vi "demo.vi"() -> ()   [LabVIEW 2016]
uses:
  test/apis/Stimulus/Helper/Helper-SubPanel/Helper-SubPanel.vi
  main/apis/Stimulus/ValueSignalByPathString.vi
  <vilib>/addons/_JKI Toolkits/Caraya/classes/Test/Test.lvclass
  test/apis/Stimulus/test_ValueSignal.lvlib
panel:
  out "error out":errorcluster
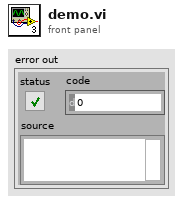
[diagram p1: front panel]
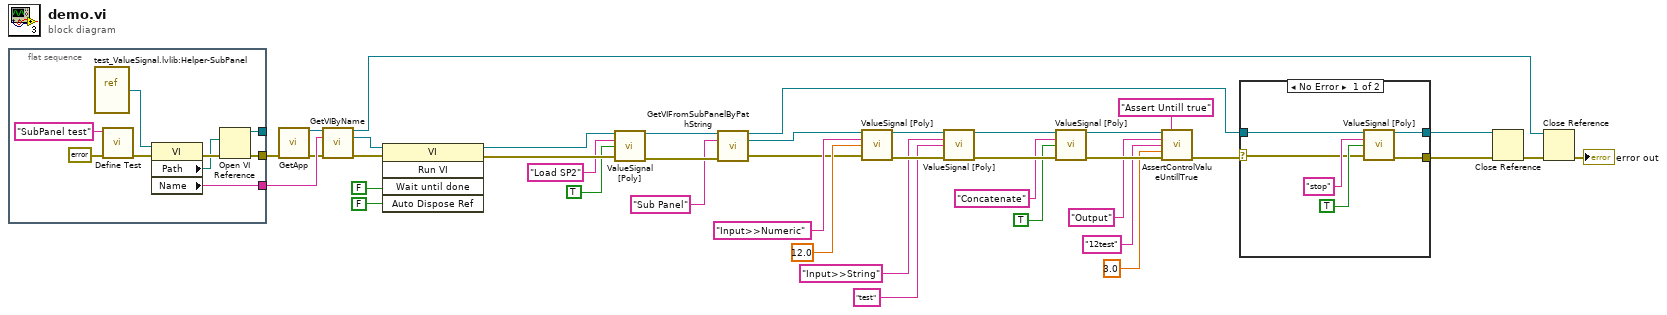
[diagram p0: block diagram]
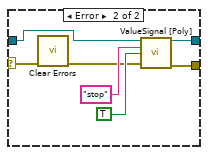
[diagram p2: hidden frame]
diagram:
  n1 = flat-sequence {
    tunnel: [w45] -> w39
    tunnel: [w44] -> _
    tunnel: [w42] -> w38
    frame #0 {
      n2 = vi-ref "test_ValueSignal.lvlib:Helper-SubPanel.vi"() -> (w47:refnum<vi>)
      n3 = call <vilib>:"Define Test.vi"("error in (no error)"=errorcluster {"status"=FALSE, "code"=0, "source"=""}, "Label (VI Title)"="SubPanel test") -> ("error out"=w48:errorcluster)  [unwired: 9 in]
      n4 = property on="Property Node" class="VI"(reference=w47, error in=w48) -> (error out=w46:errorcluster, "Path"=w43:path, "Name"=w42:string)  [unwired: 1 out]
      n5 = Open VI Reference(vi path=w43, error in (no error)=w46) -> (vi reference=w44:refnum<vi>, error out=w45:errorcluster)  [unwired: 4 in]
    }
  }
  n6 = call "GetApp.vi"("error in (no error)"=w39) -> ("Application Ref"=w40:refnum<vi>, "error out"=w37:errorcluster)  [unwired: 13 in]
  n7 = call "GetVIByName.vi"("Application Ref in"=w40, "VI Name"=w38, "error in (no error)"=w37) -> ("Application Ref out"=w36:refnum<vi>, "VI Reference"=w32:refnum<vi>, "error out"=w29:errorcluster)  [unwired: 10 in]
  n8 = invoke on="Invoke Node" class="VI" method="Run VI"(reference=w32, error in=w29, "Wait until done"=FALSE ("Wait Until Done"), "Auto Dispose Ref"=FALSE ("Auto Dispose Reference")) -> (reference out=w17:refnum<vi>, error out=w33:errorcluster)  [unwired: 1 in, 3 out]
  n9 = call-poly "ValueSignal [Poly].vi"("VI Reference In"=w17, "Control Name"="Load SP2" ("Class Name"), "Value (Signaling)"=TRUE, "error in"=w33) -> ("VI Reference Out"=w8:refnum<vi>, "error out"=w9:errorcluster)  [unwired: 10 in]
  n10 = call "GetVIFromSubPanelByPathString.vi"("VI Reference In"=w8, "SubPanel Path"="Sub Panel", "error in"=w9) -> ("VI Reference Out"=w3:refnum<vi>, "SubPanel VI Reference"=w6:refnum<vi>, "error out"=w7:errorcluster)  [unwired: 10 in]
  n11 = call-poly "ValueSignal [Poly].vi"("VI Reference In"=w6, "Control Name"="Input>>Numeric", "Value (Signaling)"=12.0, "error in"=w7) -> ("VI Reference Out"=w23:refnum<vi>, "error out"=w24:errorcluster)  [unwired: 10 in]
  n12 = call-poly "ValueSignal [Poly].vi"("VI Reference In"=w23, "Control Name"="Input>>String", "Value (Signaling)"="test" ("Control Name"), "error in"=w24) -> ("VI Reference Out"=w20:refnum<vi>, "error out"=w21:errorcluster)  [unwired: 10 in]
  n13 = call-poly "ValueSignal [Poly].vi"("VI Reference In"=w20, "Control Name"="Concatenate", "Value (Signaling)"=TRUE, "error in"=w21) -> ("VI Reference Out"=w14:refnum<vi>, "error out"=w15:errorcluster)  [unwired: 10 in]
  n14 = call "AssertControlValueUntillTrue.vi"("VI Reference In"=w14, "Label"="Assert Untill true", "Control Name"="Output", "X"="12test" ("Control Name"), "Timeout(sec)"=3.0, "error out"=w15) -> ("error out 2"=w2:errorcluster)  [unwired: 8 in, 1 out]
  n15 = case shown="No Error" w2 {
    selector: w2 -> [w51 w59]
    tunnel: [w53 w60] -> w31
    tunnel: [w52 w56] -> w30
    tunnel: w3 -> [w50 w57]
    frame No Error {
      n16 = call-poly "ValueSignal [Poly].vi"("VI Reference In"=w50, "Control Name"="stop" ("Class Name"), "Value (Signaling)"=TRUE, "error in"=w51) -> ("VI Reference Out"=w52:refnum<vi>, "error out"=w53:errorcluster)  [unwired: 10 in]
    }
    frame Error {
      n17 = call <vilib>:"Clear Errors.vi"("error in (no error)"=w59) -> ("error out"=w58:errorcluster)  [unwired: 5 in, 1 out]
      n18 = call-poly "ValueSignal [Poly].vi"("VI Reference In"=w57, "Control Name"="stop" ("Class Name"), "Value (Signaling)"=TRUE, "error in"=w58) -> ("VI Reference Out"=w56:refnum<vi>, "error out"=w60:errorcluster)  [unwired: 10 in]
    }
  }
  n19 = Close Reference(reference=w30, error in (no error)=w31) -> (error out=w35:errorcluster)
  n20 = Close Reference(reference=w36, error in (no error)=w35) -> (error out=→"error out":errorcluster)
